vi "Example Bundler Unbundler 1.vi"() -> ()   [LabVIEW 2014]
panel:
  out "Error Out":errorcluster
  in  "Error In":errorcluster
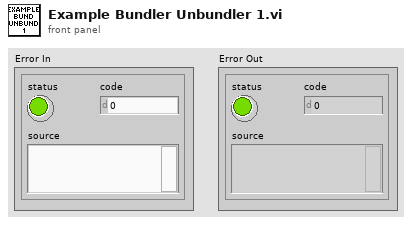
[diagram p1: front panel]
types:
  T1 = cluster{"senseOfLife":i32, "partOfBookText":string}
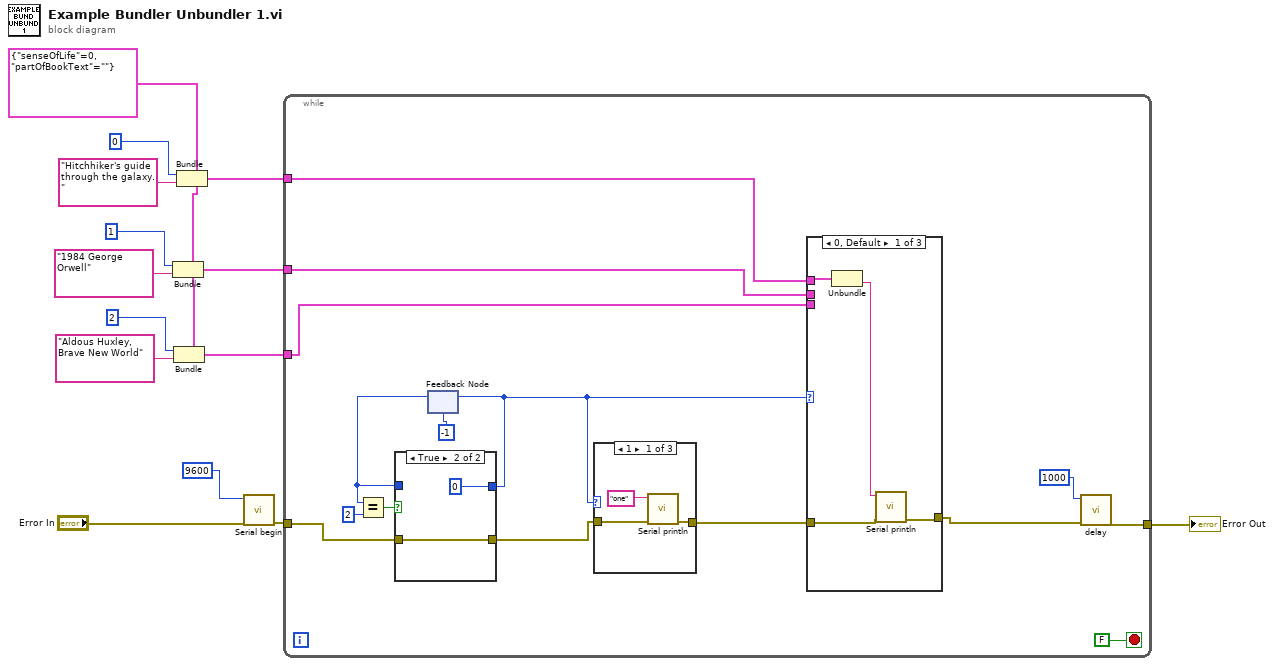
[diagram p0: block diagram]
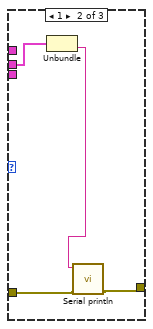
[diagram p2: hidden frame]
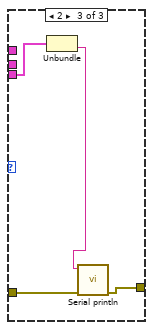
[diagram p3: hidden frame]
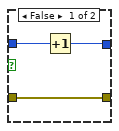
[diagram p4: hidden frame]
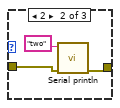
[diagram p5: hidden frame]
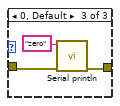
[diagram p6: hidden frame]
diagram:
  w6 = T1 {"senseOfLife"=0, "partOfBookText"=""}
  n1 = Bundle(cluster=w6, "senseOfLife"=1, "partOfBookText"="1984 George Orwell") -> (w4:T1)
  n2 = Bundle(cluster=w6, "senseOfLife"=2, "partOfBookText"="Aldous Huxley, Brave New World") -> (w3:T1)
  n3 = Bundle(cluster=w6, "senseOfLife"=0, "partOfBookText"="Hitchhiker's guide through the galaxy.") -> (w5:T1)
  n4 = call "Serial begin.vi"("Error In"="Error In", "speed (Bd)"=u16 9600 ("Baudrate")) -> ("Error Out"=w2:errorcluster)  [unwired: 9 in]
  n5 = while {
    tunnel: w2 -> [w21]
    tunnel: [w28] -> w11
    tunnel: w5 -> [w20]
    tunnel: w4 -> [w19]
    tunnel: w3 -> [w18]
    stop <- FALSE stop-if-true
    n6 = feedback #1(-1 ("senseOfLife")) -> (w23:i32)
    n7 = Equal?(x=w23, y=2 ("senseOfLife")) -> (x = y?=w25:bool)
    n8 = case shown="True" w25 {
      tunnel: [w43 0 ("senseOfLife")] -> w17
      tunnel: w23 -> [w44 _]
      tunnel: [w42 w45] -> w22
      tunnel: w21 -> [w42 w45]
      frame False {
        n9 = Increment(x=w44) -> (x+1=w43:i32)
      }
      frame True {
      }
    }
    n10 = feedback-in #1(w17) -> ()
    n11 = case shown="1" w17 {
      tunnel: w22 -> [w49 w51 w53]
      tunnel: [w48 w52 w55] -> w16
      frame 1 {
        n12 = call "Serial println.vi"("Error In"=w49, "string in"="one" ("String to print")) -> ("Error Out"=w48:errorcluster)  [unwired: 9 in]
      }
      frame 2 {
        n13 = call "Serial println.vi"("Error In"=w51, "string in"="two" ("String to print")) -> ("Error Out"=w52:errorcluster)  [unwired: 9 in]
      }
      frame 0, Default {
        n14 = call "Serial println.vi"("Error In"=w53, "string in"="zero" ("String to print")) -> ("Error Out"=w55:errorcluster)  [unwired: 9 in]
      }
    }
    n15 = case shown="0, Default" w17 {
      tunnel: w16 -> [w31 w36 w39]
      tunnel: w20 -> [w33 _ _]
      tunnel: w19 -> [_ w37 _]
      tunnel: w18 -> [_ _ w41]
      tunnel: [w32 w35 w40] -> w15
      frame 0, Default {
        n16 = Unbundle(w33) -> ("partOfBookText"=w30:string)  [unwired: 1 out]
        n17 = call "Serial println.vi"("Error In"=w31, "string in"=w30) -> ("Error Out"=w32:errorcluster)  [unwired: 9 in]
      }
      frame 1 {
        n18 = Unbundle(w37) -> ("partOfBookText"=w34:string)  [unwired: 1 out]
        n19 = call "Serial println.vi"("Error In"=w36, "string in"=w34) -> ("Error Out"=w35:errorcluster)  [unwired: 9 in]
      }
      frame 2 {
        n20 = Unbundle(w41) -> ("partOfBookText"=w38:string)  [unwired: 1 out]
        n21 = call "Serial println.vi"("Error In"=w39, "string in"=w38) -> ("Error Out"=w40:errorcluster)  [unwired: 9 in]
      }
    }
    n22 = call "delay.vi"("Error In"=w15, "time (ms)"=1000) -> ("Error Out"=w28:errorcluster)  [unwired: 9 in]
  }
  "Error Out" <- w11
